vi "FPGA Wait On IRQs.vi"(6 "Timeout (ms)":u32=5000, 8 "error in (no error)":errorcluster, 10 "IRQs":u32[](array[numeric]), 11 "FPGA Session In":refnum<class "FPGA Interface Base.lvclass">) -> (0 "error out":errorcluster, 2 "IRQs Asserted":u32[](array[numeric]), 3 "FPGA Session Out":refnum<class "FPGA Interface Base.lvclass">, 4 "Timed Out?":bool)   [LabVIEW 2010, in "FPGA Interface Base.lvclass"]
doc: "This is a blocking function that stops the calling thread until the FPGA asserts any IRQ in the irqs parameter, or until the function call times out. Before calling this function, you must use NiFpga_ReserveIrqContext to reserve an IRQ context. No other threads can use the same context when this function is called. You can use the irqsAsserted parameter to determine which IRQs were asserted for each function call."
uses:
  <userlib>/_FPGA Interface Advanced Tools/FPGA Interface Base/FPGA Interface Base.lvclass
  <userlib>/_FPGA Interface Advanced Tools/FPGA Interface Base/Accessors/FPGA Read Session.vi
  <userlib>/_FPGA Interface Advanced Tools/FPGA Interface Base/Accessors/FPGA Read IRQ Context Queue.vi
  <vilib>/Utility/error.llb/Error Cluster From Error Code.vi
  <userlib>/_FPGA Interface Advanced Tools/FPGA Interface Wrapper/FPGA Interface Wrapper.lvlib
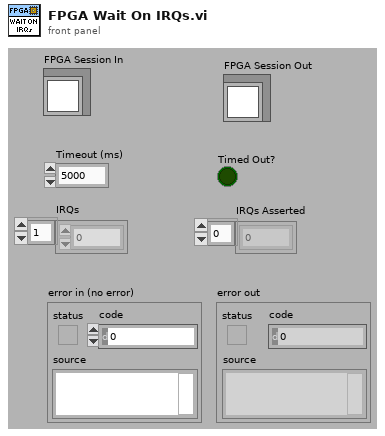
[diagram p1: front panel]
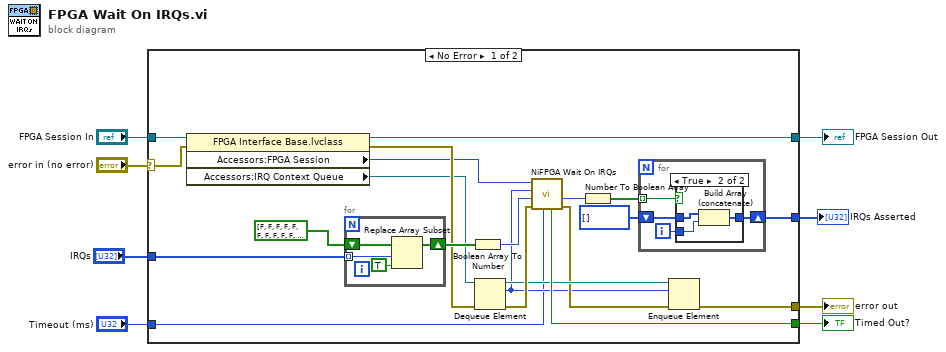
[diagram p0: block diagram]
diagram:
  n1 = case shown="No Error" "error in (no error)" {
    selector: "error in (no error)" -> [w13 w43]
    tunnel: [w17 w43] -> w4
    tunnel: [w9 w42] -> w7
    tunnel: "FPGA Session In" -> [w14 w42]
    tunnel: "IRQs" -> [w24 _]
    tunnel: [w21 _] -> w2
    tunnel: [w28 _] -> w5
    tunnel: "Timeout (ms)" -> [w15 _]
    frame No Error {
      n2 = property class="FPGA Interface Base.lvclass"(reference=w14, error in=w13) -> (reference out=w9:refnum<class "FPGA Interface Base.lvclass">, error out=w12:errorcluster, "Accessors:FPGA Session"=w10:u32, "Accessors:IRQ Context Queue"=w11:refnum<queue>)
      n3 = for {
        tunnel: w24 -> [w40] mode=indexing
        shift-right: [w38] -> w26
        shift-left: bool[] [FALSE, FALSE, FALSE, FALSE, FALSE, FALSE, FALSE, FALSE, FALSE, FALSE, FALSE, FALSE, FALSE, FALSE, FALSE, FALSE, FALSE, FALSE, FALSE, FALSE, FALSE, FALSE, FALSE, FALSE, FALSE, FALSE, FALSE, FALSE, FALSE, FALSE, FALSE, FALSE] -> [w41]
        n4 = Replace Array Subset(array=w41, new element=TRUE ("new element/subarray"), index=w40) -> (w38:bool[])
      }
      n5 = Boolean Array To Number(Boolean array=w26) -> (number=w23:u32)
      n6 = Dequeue Element(queue=w11, error in (no error)=w12) -> (queue out=w20:refnum<queue>, element=w18:u32, error out=w27:errorcluster)  [unwired: 1 in, 1 out]
      n7 = call <userlib>:"NiFPGA Wait On IRQs.vi"("Timeout"=w15, "error in (no error)"=w27, "IRQs"=w23, "Context"=w18, "Session In"=w10) -> ("error out"=w19:errorcluster, "IRQs Asserted"=w29:u32, "Timed Out?"=w28:bool)  [unwired: 3 in, 1 out]
      n8 = Number To Boolean Array(number=w29) -> (Boolean array=w22:bool[])
      n9 = for {
        tunnel: w22 -> [w32] mode=indexing
        shift-right: [w31] -> w21
        shift-left: u32[] [] -> [w30]
        i -> [w33]
        n10 = case shown="True" w32 {
          tunnel: w33 -> [_ w35]
          tunnel: [w34 w37] -> w31
          tunnel: w30 -> [w34 w36]
          frame False {
          }
          frame True {
            n11 = Build Array (concatenate)(w36, w35) -> (w37:u32[])
          }
        }
      }
      n12 = Enqueue Element(queue=w20, element=w18, error in (no error)=w19) -> (error out=w17:errorcluster)  [unwired: 1 in, 2 out]
    }
    frame Error {
    }
  }
  "error out" <- w4
  "Timed Out?" <- w5
  "FPGA Session Out" <- w7
  "IRQs Asserted" <- w2
